vi "feedback node.vi"() -> ()   [LabVIEW 2022 SP3]
panel:
  out "x*y":i32
  in  "Numeric 3":i32
  out "Numeric 2":i32
  in  "Numeric":i32
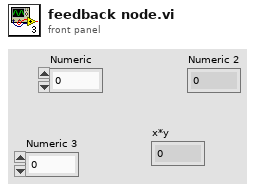
[diagram p1: front panel]
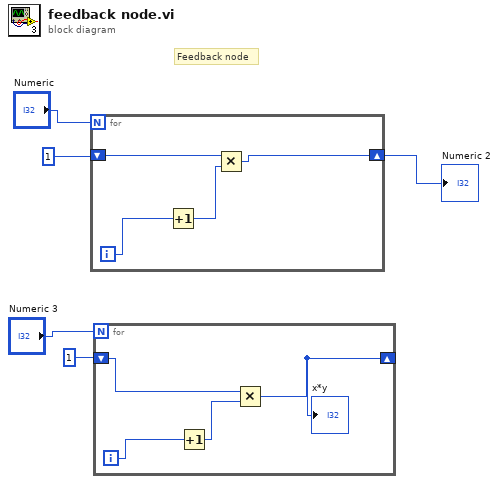
[diagram p0: block diagram]
diagram:
  # "Feedback node"
  n1 = for {
    N: "Numeric" -> [_]
    shift-right: [w6] -> w3
    shift-left: 1 -> [w9]
    i -> [w8]
    n2 = Increment(x=w8) -> (x+1=w7:i32)
    n3 = Multiply(x=w9, y=w7) -> (x*y=w6:i32)
  }
  "Numeric 2" <- w3
  n4 = for {
    N: "Numeric 3" -> [_]
    shift-right: [w10] -> _
    shift-left: 1 -> [w11]
    i -> [w13]
    n5 = Increment(x=w13) -> (x+1=w12:i32)
    n6 = Multiply(x=w11, y=w12) -> (x*y=w10:i32)
    "x*y" <- w10
  }
